vi "get incoming object Information element by name.vi"(10 "name":string, 11 "interaction_attribute_type":T1) -> (1 "found":bool, 3 "element out":dbl)   [LabVIEW 2019, in "HLA Custom Device Engine.lvlib"]
uses:
  HLA Custom Device Engine.lvlib
  _typedefs/object_info_received_type.ctl
  <vilib>/addons/hla/TransportationType.ctl
  <vilib>/addons/hla/OrderType.ctl
  <vilib>/addons/hla/openrti_rti1516eLv.lvlib
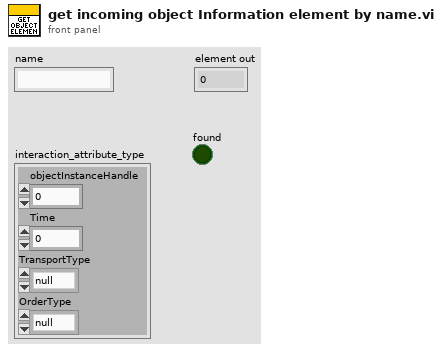
[diagram p1: front panel]
types:
  T1 = typedef "HLA Custom Device Engine.lvlib/object_info_received_type.ctl" = cluster{"objectInstanceHandle":u64, "Time":dbl, "TransportType":T2, "OrderType":T3}
  T2 = typedef "openrti_rti1516eLv.lvlib/TransportationType.ctl" = enum32{"null", "RELIABLE", "BEST_EFFORT"}
  T3 = typedef "openrti_rti1516eLv.lvlib/OrderType.ctl" = enum32{"null", "RECEIVE", "TIMESTAMP"}
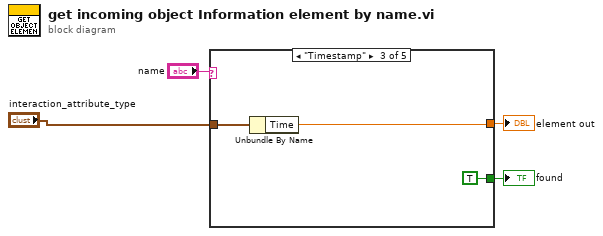
[diagram p0: block diagram]
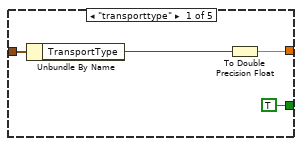
[diagram p2: hidden frame]
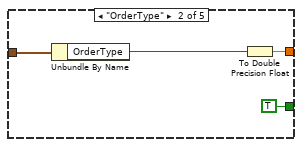
[diagram p3: hidden frame]
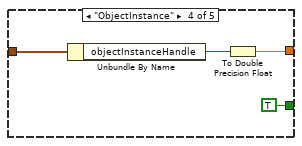
[diagram p4: hidden frame]
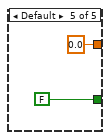
[diagram p5: hidden frame]
diagram:
  n1 = case shown="\"Timestamp\"" "name" {
    tunnel: "interaction_attribute_type" -> [w7 w12 w14 w19 _]
    tunnel: [w6 w11 w15 w18 0.0] -> w2
    tunnel: [TRUE TRUE TRUE TRUE FALSE] -> w1
    frame "transporttype" {
      n2 = Unbundle By Name(w7) -> ("TransportType"=w8:T2)
      n3 = To Double Precision Float(number=w8) -> (double precision float=w6:dbl)
    }
    frame "OrderType" {
      n4 = Unbundle By Name(w12) -> ("OrderType"=w10:T3)
      n5 = To Double Precision Float(number=w10) -> (double precision float=w11:dbl)
    }
    frame "Timestamp" {
      n6 = Unbundle By Name(w14) -> ("Time"=w15:dbl)
    }
    frame "ObjectInstance" {
      n7 = Unbundle By Name(w19) -> ("objectInstanceHandle"=w16:u64)
      n8 = To Double Precision Float(number=w16) -> (double precision float=w18:dbl)
    }
    frame Default {
    }
  }
  "element out" <- w2
  "found" <- w1
